vi "GoalieNormal.vi"(8 "Robot":T1={"id"=0, "function"=enum."Attacker", "x"=0.0, "y"=0.0, "orientation"=0.0, "v_tangent"=0.0, "v_normal"=0.0, "v_ang"=0.0, "kick_x"=0.0, "kick_z"=0.0, "dribble"=FALSE, "Timestamp"=timestamp(0 s since 1904-01-01), "dest_x"=0.0, "dest_y"=0.0, "dest_orientation"=0.0, "estimatives"={"est_v_tangent"=0.0, "est_v_normal"=0.0, "est_vx"=0.0, "est_vy"=0.0}, "dest_x_kick"=0.0, "dest_y_kick"=0.0, "Gap Coord"=[], "States"=enum."GoToTangent"}, 11 "IA Input":T4={"our_robots"=[], "enemy_robots"=[], "balls"=[], "geometry"={"line_width"=0, "field_length"=0, "field_width"=0, "boundary_width"=0, "referee_width"=0, "goal_width"=0, "goal_depth"=0, "goal_wall_width"=0, "center_circle_radius"=0, "defense_radius"=0, "defense_stretch"=0, "free_kick_from_defense_dist"=0, "penalty_spot_from_field_line_dist"=0, "penalty_line_from_spot_dist"=0}, "IA Judge"={"stage"="", "command"="", "our_goalie_id"=0.0, "enemy_goalie_id"=0.0, "command\nenum"=enum."Halt", "Time"=enum."Azul"}, "Received Timestamp"=timestamp(0 s since 1904-01-01), "Events"={"Touch"=FALSE, "Ball out"=FALSE, "id touch"=0.0, "Ball out of \nVision"=FALSE, "Ball inside \nGoalie area"=FALSE, "Robot not responding"=FALSE, "Robots responding status"=[1.0, 1.0, 1.0, 1.0, 1.0, 1.0], "Enemy Ball \nPossession"=FALSE}}) -> (2 "output cluster":T1={"id"=0, "function"=enum."Attacker", "x"=0.0, "y"=0.0, "orientation"=0.0, "v_tangent"=0.0, "v_normal"=0.0, "v_ang"=0.0, "kick_x"=0.0, "kick_z"=0.0, "dribble"=FALSE, "Timestamp"=timestamp(0 s since 1904-01-01), "dest_x"=0.0, "dest_y"=0.0, "dest_orientation"=0.0, "estimatives"={"est_v_tangent"=0.0, "est_v_normal"=0.0, "est_vx"=0.0, "est_vy"=0.0}, "dest_x_kick"=0.0, "dest_y_kick"=0.0, "Gap Coord"=[], "States"=enum."GoToTangent"})   [LabVIEW 2016]
uses:
  Core/AI Input.ctl
  Core/AI Robot.ctl
  Functions Enum.ctl
  AttackerStates.ctl
  Core/AI Ball.ctl
  Core/Field Size.ctl
  Core/AI Judge.ctl
  Command Enum.ctl
panel:
  in  "Time kick (s)":dbl=1.0 caption="Time Target (s)"
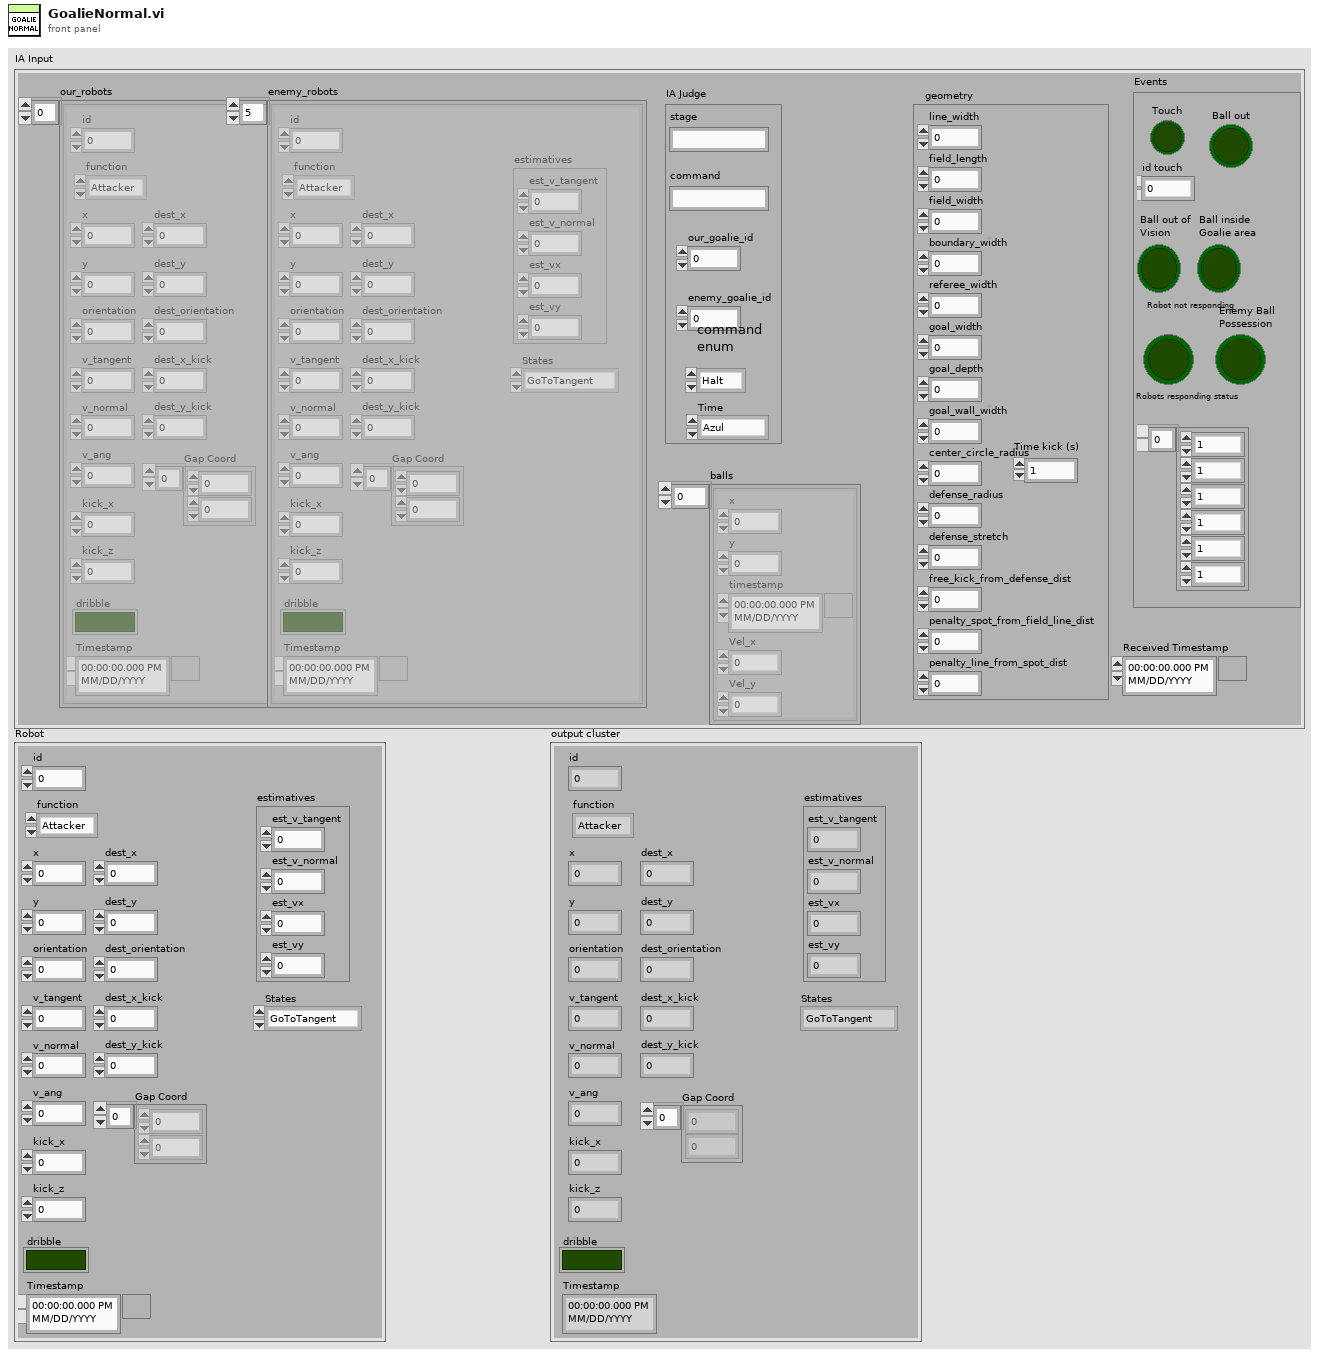
[diagram p1: front panel]
types:
  T1 = typedef "AI Robot.ctl" = cluster{"id":u32, "function":T2, "x":dbl, "y":dbl, "orientation":dbl, "v_tangent":dbl, "v_normal":dbl, "v_ang":dbl, "kick_x":dbl, "kick_z":dbl, "dribble":bool, "Timestamp":timestamp, "dest_x":dbl, "dest_y":dbl, "dest_orientation":dbl, "estimatives":cluster{"est_v_tangent":dbl, "est_v_normal":dbl, "est_vx":dbl, "est_vy":dbl}, "dest_x_kick":dbl, "dest_y_kick":dbl, "Gap Coord":dbl[], "States":T3}
  T2 = typedef "Functions Enum.ctl" = enum16{"Attacker", "Goalie", "Defender", "Striker", "Goto 0", "Dummy", "Kicker", "ZigZag"}
  T3 = typedef "AttackerStates.ctl" = enum16{"Pass", "GoToTangent", "BallGetting", "GoToKick", ""}
  T4 = typedef "AI Input.ctl" = cluster{"our_robots":T1[], "enemy_robots":T1[], "balls":T5[], "geometry":T6, "IA Judge":T7, "Received Timestamp":timestamp, "Events":cluster{"Touch":bool, "Ball out":bool, "id touch":dbl, "Ball out of \nVision":bool, "Ball inside \nGoalie area":bool, "Robot not responding":bool, "Robots responding status":dbl[], "Enemy Ball \nPossession":bool}}
  T5 = typedef "AI Ball.ctl" = cluster{"x":dbl, "y":dbl, "timestamp":timestamp, "Vel_x":dbl, "Vel_y":dbl}
  T6 = typedef "Field Size.ctl" = cluster{"line_width":u32, "field_length":u32, "field_width":u32, "boundary_width":u32, "referee_width":u32, "goal_width":u32, "goal_depth":u32, "goal_wall_width":u32, "center_circle_radius":u32, "defense_radius":u32, "defense_stretch":u32, "free_kick_from_defense_dist":u32, "penalty_spot_from_field_line_dist":u32, "penalty_line_from_spot_dist":u32}
  T7 = typedef "AI Judge.ctl" = cluster{"stage":string, "command":string, "our_goalie_id":dbl, "enemy_goalie_id":dbl, "command\nenum":T8, "Time":enum16{"Azul", "Amarelo"}}
  T8 = typedef "Command Enum.ctl" = enum16{"Halt", "Stop", "Force Start", "PKA Normal Start", "Prepare Kickoff Ally", "PKE Normal Start", "Prepare Kickoff Enemy", "Prepare Penalty Ally", "PPA Normal Start", "Prepare Penalty Enemy", "PPE Normal Start", "Direct Free Enemy", "Direct Free Ally", "Indirect Free Enemy", "Indirect Free Ally", "Timeout Enemy", "Timeout Ally", "Goal Enemy", "Goal Ally", "Ball Placement Enemy", "Ball Placement Ally", "Normal Half Time", "Extra Time Break", "Extra Half Time", "None"}
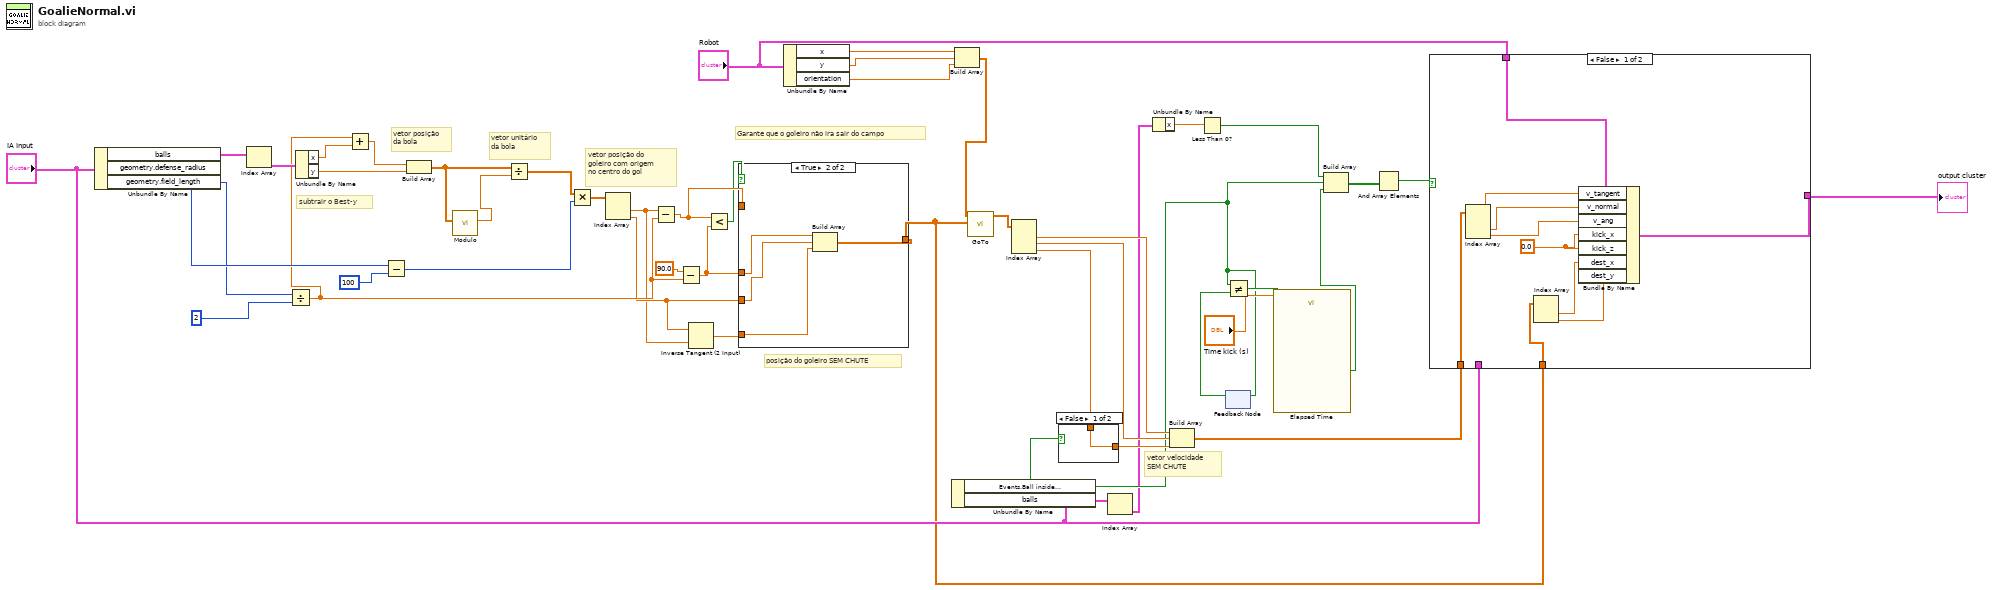
[diagram p0: block diagram]
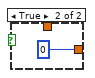
[diagram p2: hidden frame]
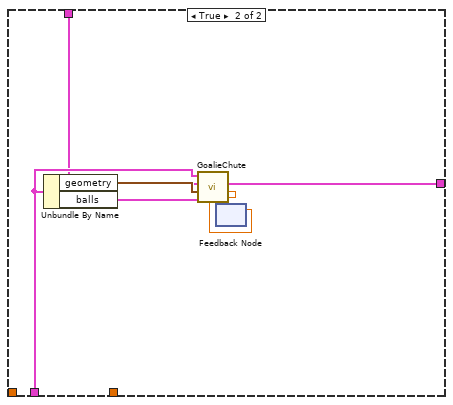
[diagram p3: hidden frame]
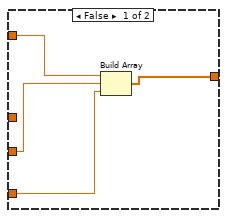
[diagram p4: hidden frame]
diagram:
  # "vetor velocidade SEM CHUTE"
  # "posição do goleiro SEM CHUTE"
  # "Garante que o goleiro não ira sair do campo"
  # "vetor posição do goleiro com origem no centro do gol"
  # "subtrair o Best-y"
  # "vetor unitário da bola"
  # "vetor posição da bola"
  n1 = Unbundle By Name("IA Input") -> ("balls"=w47:T5[], "geometry.defense_radius"=w42:u32, "geometry.field_length"=w26:u32)
  n2 = Index Array(array=w47) -> (element=w46:T5)  [unwired: 1 in]
  n3 = Divide(x=w26, y=u32 2) -> (x/y=w25:dbl)
  n4 = Unbundle By Name(w46) -> ("x"=w27:dbl, "y"=w28:dbl)
  n5 = Add(x=w25, y=w27) -> (x+y=w24:dbl)
  n6 = Subtract(x=w42, y=u32 100) -> (x-y=w41:u32)
  n7 = Build Array(w24, w28) -> (w45:dbl[])
  n8 = call "Modulo.vi"("2D vector"=w45) -> ("Modulo"=w44:dbl)  [unwired: 10 in]
  n9 = Divide(x=w45, y=w44) -> (x/y=w43:dbl[])
  n10 = Multiply(x=w43, y=w41) -> (x*y=w39:dbl[])
  n11 = Index Array(array=w39) -> (element #1=w22:dbl, element #2=w23:dbl)  [unwired: 2 in]
  n12 = Subtract(x=w22, y=w25) -> (x-y=w35:dbl)
  n13 = Subtract(x=90.0, y=w25) -> (x-y=w36:dbl)
  n14 = Inverse Tangent (2 Input)(1:w22, 2:w23) -> (0:w21:dbl)
  n15 = Less?(x=w35, y=w36) -> (x < y?=w29:bool)
  n16 = case shown="True" w29 {
    tunnel: w23 -> [w50 w53]
    tunnel: w36 -> [_ w55]
    tunnel: w35 -> [w51 _]
    tunnel: [w49 w54] -> w1
    tunnel: w21 -> [w48 w52]
    frame False {
      n17 = Build Array(w51, w50, w48) -> (w49:dbl[])
    }
    frame True {
      n18 = Build Array(w55, w53, w52) -> (w54:dbl[])
    }
  }
  n19 = Unbundle By Name("Robot") -> ("x"=w34:dbl, "y"=w33:dbl, "orientation"=w32:dbl)
  n20 = Unbundle By Name("IA Input") -> ("Events.Ball inside \nGoalie area"=w8:bool, "balls"=w5:T5[])
  n21 = Build Array(w34, w33, w32) -> (w31:dbl[])
  n22 = call "GoTo.vi"("Target"=w1, "Position"=w31) -> ("Output\nVelocity"=w30:dbl[])  [unwired: 8 in, 1 out]
  n23 = Index Array(array=w30) -> (element #1=w15:dbl, element #2=w16:dbl, element #3=w17:dbl)  [unwired: 3 in]
  n24 = case shown="False" w8 {
    tunnel: [w56 0] -> w18
    tunnel: w17 -> [w56 _]
    frame False {
    }
    frame True {
    }
  }
  n25 = Index Array(array=w5) -> (element=w4:T5)  [unwired: 1 in]
  n26 = Unbundle By Name(w4) -> ("x"=w3:dbl)
  n27 = Build Array(w15, w16, w18) -> (w13:dbl[])
  n28 = Less Than 0?(x=w3) -> (x < 0?=w2:bool)
  n29 = feedback #1() -> (w9:bool)  [unwired: 1 in]
  n30 = feedback-in #1(w8) -> ()
  n31 = Not Equal?(x=w8, y=w9) -> (x != y?=w11:bool)
  n32 = call "Elapsed Time"("Time Target (s)"="Time kick (s)", "Reset"=w11) -> ("Time has Elapsed"=w10:bool)  [unwired: 10 in, 7 out]
  n33 = Build Array(w2, w8, w10) -> (w6:bool[])
  n34 = And Array Elements(Boolean array=w6) -> (logical AND=w7:bool)
  n35 = case shown="False" w7 {
    tunnel: "IA Input" -> [_ w74]
    tunnel: "Robot" -> [w67 w72]
    tunnel: [w66 w68] -> w14
    tunnel: w13 -> [w64 _]
    tunnel: w1 -> [w60 _]
    frame False {
      w65 = 0.0 ("kick_z")
      n36 = Index Array(array=w64) -> (element #1=w63:dbl, element #2=w62:dbl, element #3=w61:dbl)  [unwired: 3 in]
      n37 = Index Array(array=w60) -> (element #1=w59:dbl, element #2=w58:dbl)  [unwired: 2 in]
      n38 = Bundle By Name(cluster=w67, "v_tangent"=w63, "v_normal"=w62, "v_ang"=w61, "kick_x"=w65, "kick_z"=w65, "dest_x"=w59, "dest_y"=w58) -> (w66:T1)
    }
    frame True {
      n39 = Unbundle By Name(w74) -> ("geometry"=w73:T6, "balls"=w71:T5[])
      n40 = feedback #2() -> (w69:dbl)  [unwired: 1 in]
      n41 = call "GoalieChute.vi"("Current State"=w69, "balls"=w71, "Field Size in"=w73, "Robot in"=w72, "IA State Input 2"=w74) -> ("Next State"=w70:dbl, "Robot out"=w68:T1)  [unwired: 5 in]
      n42 = feedback-in #2(w70) -> ()
    }
  }
  "output cluster" <- w14
